vi "Vehicle out of Position Update.vi"(8 "error in (no error)":errorcluster, 10 "Vehicle ouf ot Position":bool, 11 "Normal Car Position Simulation View in":refnum<class "Normal Car Position Simulation View.lvclass">) -> (0 "error out":errorcluster, 3 "Normal Car Position Simulation View out":refnum<class "Normal Car Position Simulation View.lvclass">)   [LabVIEW 2019, in "Normal Car Position Simulation View.lvclass"]
uses:
  <vilib>/gpm_packages/@cs/Car-wash/Source/Normal Car Position Simulation View/Normal Car Position Simulation View/Normal Car Position Simulation View.lvclass
  C:/Program Files/National Instruments/LabVIEW 2019/vi.lib/gpm_packages/@cs/Car-wash/Source/Car Position Simulation View Definition/Car Position Simulation View Definition/Car Position Simulation View Definition.lvclass
  <vilib>/gpm_packages/@cs/Car-wash/Source/Car Position Simulation View Definition/Car Position Simulation View Definition/Car Position Simulation View Definition.lvclass/Car Position Simulation View Definition.ctl
  <vilib>/gpm_packages/@cs/Car-wash/Source/Car Position Simulation View Definition/Car Position Simulation View Definition/Car Position Simulation View Definition.lvclass
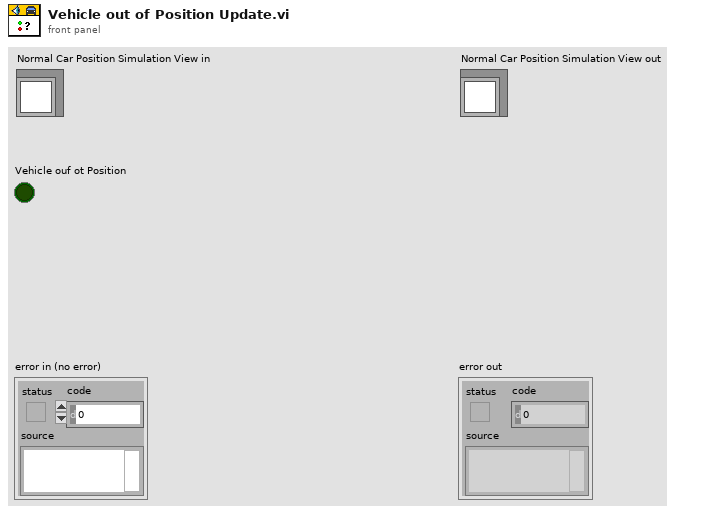
[diagram p1: front panel]
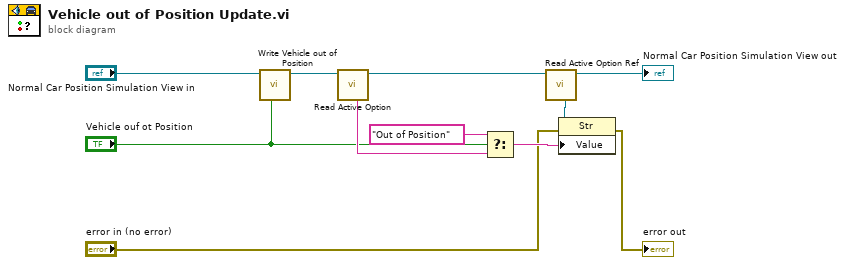
[diagram p0: block diagram]
diagram:
  n1 = call <vilib>:"Write Vehicle out of Position.vi"("Vehicle out of Position"="Vehicle ouf ot Position", "Car Position Simulation View Definition in"="Normal Car Position Simulation View in") -> ("Car Position Simulation View Definition out"=w2:refnum<class "Normal Car Position Simulation View.lvclass">)  [unwired: 9 in]
  n2 = call <vilib>:"Read Active Option.vi"("Car Position Simulation View Definition in"=w2) -> ("Car Position Simulation View Definition out"=w11:refnum<class "Normal Car Position Simulation View.lvclass">, "Active Option"=w9:string)  [unwired: 9 in]
  n3 = Select(t="Out of Position", s="Vehicle ouf ot Position", f=w9) -> (s? t:f=w7:string)
  n4 = call <vilib>:"Read Active Option Ref.vi"("Car Position Simulation View Definition in"=w11) -> ("Car Position Simulation View Definition out"=→"Normal Car Position Simulation View out":refnum<class "Normal Car Position Simulation View.lvclass">, "Active Option Ref"=w10:refnum<vi>)  [unwired: 9 in]
  n5 = property class="Str"(reference=w10, error in="error in (no error)", "Value"=w7) -> (error out=→"error out":errorcluster)  [unwired: 1 out]
